vi "WPI_DigitalModuleDIOCache.vi"(7 "Operation":T2, 8 "error in (no error)":errorcluster, 11 "DIOChannel":T1=enum."DIO 1") -> (0 "error out":errorcluster, 2 "Allocated":bool, 3 "DIOChannel Allocated":T1=enum."DIO 1")   [LabVIEW 2017]
doc: "This software is licensed. Open the labview\\readme\\WPI Robotics Library Open Source License.txt file for more information."
uses:
  <vilib>/Rock Robotics/WPI/DigitalModule/WPI_DigitalModuleDIOCacheOp.ctl
  <vilib>/Rock Robotics/SystemInterfaces/DIO/FPGA_DIOChannel.ctl
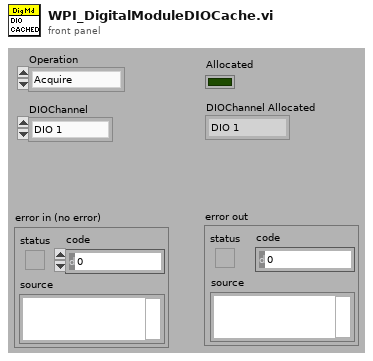
[diagram p1: front panel]
types:
  T1 = typedef "FPGA_DIOChannel.ctl" = enum8{"DIO 0", "DIO 1", "DIO 2", "DIO 3", "DIO 4", "DIO 5", "DIO 6", "DIO 7", "DIO 8", "DIO 9", "DIO MXP 0", "DIO MXP 1", "DIO MXP 2", "DIO MXP 3", "DIO MXP 4", "DIO MXP 5", "DIO MXP 6", "DIO MXP 7", "DIO MXP 8", "DIO MXP 9", "DIO MXP 10", "DIO MXP 11", "DIO MXP 12", "DIO MXP 13", "DIO MXP 14", "DIO MXP 15", "SPI Port CS1", "SPI Port CS2", "SPI Port CS3", "SPI Port MISO", "SPI Port MOSI", "Invalid"}
  T2 = typedef "WPI_DigitalModuleDIOCacheOp.ctl" = enum16{"Acquire", "Release", "Status"}
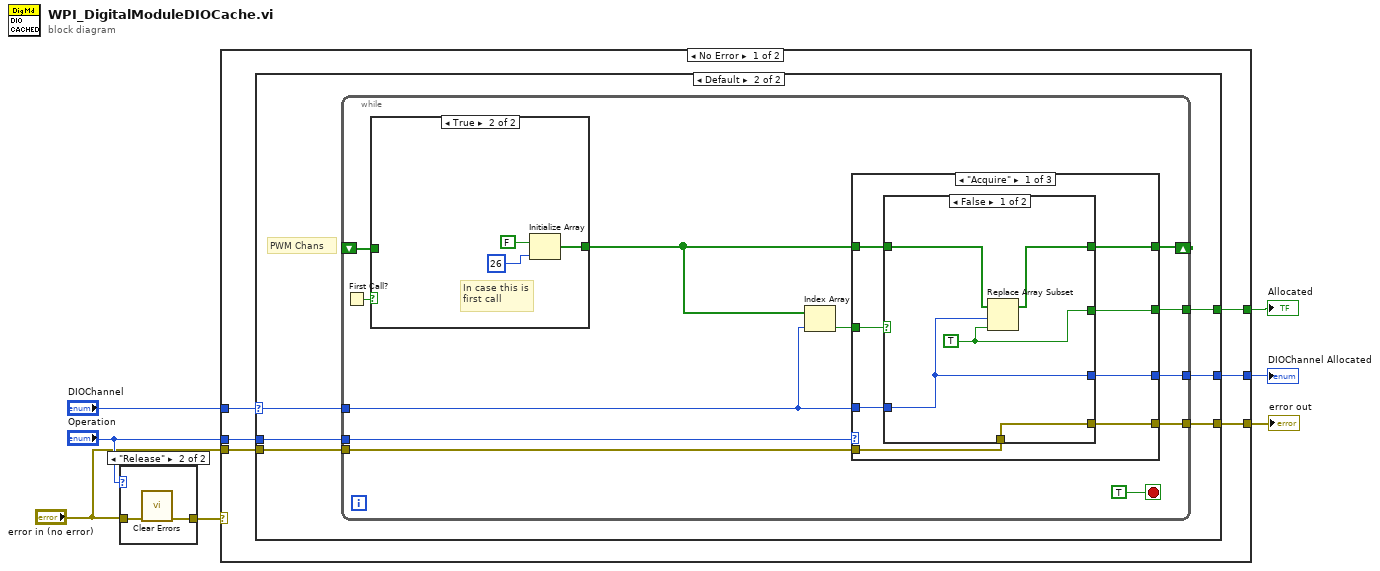
[diagram p0: block diagram]
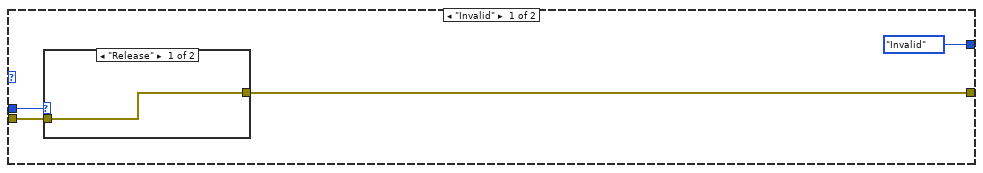
[diagram p3: hidden frame]
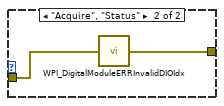
[diagram p4: hidden frame]
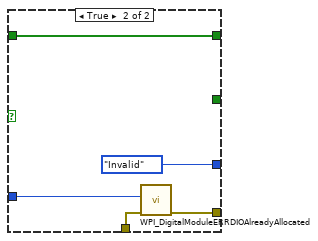
[diagram p5: hidden frame]
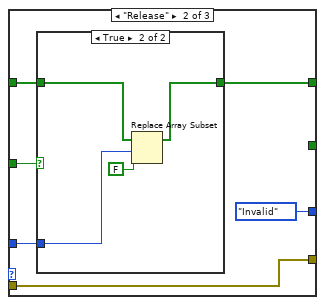
[diagram p6: hidden frame]
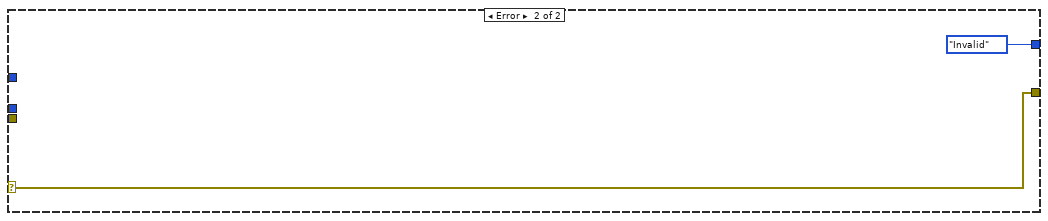
[diagram p10: hidden frame]
diagram:
  n1 = case shown="\"Release\"" "Operation" {
    tunnel: "error in (no error)" -> [w8 w10]
    tunnel: [w8 w9] -> w4
    frame "Acquire", Default {
    }
    frame "Release" {
      n2 = call <vilib>:"Clear Errors.vi"("error in (no error)"=w10) -> ("error out"=w9:errorcluster)  [unwired: 1 in, 5 out]
    }
  }
  n3 = case shown="No Error" w4 {
    selector: w4 -> [_ w80]
    tunnel: "Operation" -> [w16 _]
    tunnel: "DIOChannel" -> [w15 _]
    tunnel: [w14 w80] -> w1
    tunnel: [w13 _] -> w6
    tunnel: [w12 FPGA_DIOChannel."Invalid" ("DIOChannel Allocated")] -> w3
    tunnel: "error in (no error)" -> [w11 _]
    frame No Error {
      n4 = case shown="Default" w15 {
        selector: w15 -> [_ w25]
        tunnel: w16 -> [w20 w29]
        tunnel: [w19 w28] -> w14
        tunnel: [_ w27] -> w13
        tunnel: [FPGA_DIOChannel."Invalid" ("DIOChannel") w26] -> w12
        tunnel: w11 -> [w17 w24]
        frame "Invalid" {
          n5 = case shown="\"Release\"" w20 {
            tunnel: [w21 w23] -> w19
            tunnel: w17 -> [w21 w22]
            frame "Release" {
            }
            frame "Acquire", "Status" {
              n6 = call <vilib>:"WPI_DigitalModuleERRInvalidDIOIdx.vi"("error in (no error)"=w22) -> ("error out"=w23:errorcluster)
            }
          }
        }
        frame Default {
          # "PWM Chans"
          n7 = while {
            shift-right: [w38] -> _
            shift-left: _ -> [w40]
            tunnel: w29 -> [w39]
            tunnel: w25 -> [w34]
            tunnel: [w37] -> w28
            tunnel: [w36] -> w27
            tunnel: [w33] -> w26
            tunnel: w24 -> [w31]
            stop <- TRUE stop-if-true
            n8 = First Call?() -> (First Call?: T/F=w41:bool)
            n9 = case shown="True" w41 {
              tunnel: w40 -> [w75 _]
              tunnel: [w75 w77] -> w35
              frame False {
              }
              frame True {
                # "In case this is\nfirst call"
                n10 = Initialize Array(FALSE, 26 ("dimension size")) -> (w77:bool[])
              }
            }
            n11 = Index Array(array=w35, index=w34) -> (element=w30:bool)
            n12 = case shown="\"Acquire\"" w39 {
              tunnel: w35 -> [w45 w65 w74]
              tunnel: [w49 w63 w74] -> w38
              tunnel: w34 -> [w48 w64 w72]
              tunnel: [w47 w60 w71] -> w37
              tunnel: [w46 _ w73] -> w36
              tunnel: w30 -> [w44 w62 w73]
              tunnel: [w43 FPGA_DIOChannel."Invalid" ("DIOChannel Allocated") w72] -> w33
              tunnel: w31 -> [w42 w60 w71]
              frame "Acquire" {
                n13 = case shown="False" w44 {
                  tunnel: w45 -> [w53 w59]
                  tunnel: [w52 w59] -> w49
                  tunnel: w48 -> [w51 w55]
                  tunnel: [w50 w58] -> w47
                  tunnel: [w54 _] -> w46
                  tunnel: [w51 FPGA_DIOChannel."Invalid" ("DIOChannel Allocated")] -> w43
                  tunnel: w42 -> [w50 w56]
                  frame False {
                    w54 = TRUE ("new element/subarray")
                    n14 = Replace Array Subset(array=w53, new element=w54, index=w51) -> (w52:bool[])
                  }
                  frame True {
                    n15 = call <vilib>:"WPI_DigitalModuleERRDIOAlreadyAllocated.vi"("error in (no error)"=w56, "DIOChannel"=w55) -> ("error out"=w58:errorcluster)  [unwired: 9 in]
                  }
                }
              }
              frame "Release" {
                n16 = case shown="True" w62 {
                  tunnel: w65 -> [w66 w70]
                  tunnel: w64 -> [_ w69]
                  tunnel: [w66 w68] -> w63
                  frame False {
                  }
                  frame True {
                    n17 = Replace Array Subset(array=w70, new element=FALSE ("new element/subarray"), index=w69) -> (w68:bool[])
                  }
                }
              }
              frame "Status" {
              }
            }
          }
        }
      }
    }
    frame Error {
    }
  }
  "Allocated" <- w6
  "error out" <- w1
  "DIOChannel Allocated" <- w3
